vi "Differentiate 3D.vi"(0 "Timebase":dbl[](array[numeric]) format="%.2f", 3 "Sample Rate 4":dbl format="%.2f", 4 "Fixed Sample Rate":bool=TRUE, 5 "Data (in)":dbl[][](array[numeric]) format="%.2f") -> (2 "Data (differentiated)":dbl[][](graph))   [LabVIEW 2016]
uses:
  <vilib>/Analysis/2dsp.llb/Derivative x(t).vi
  <vilib>/Analysis/NI_AALPro.lvlib
panel:
  out "Data (differentiated) 2":dbl[][](graph)
  in  "Minimum TIme difference 1ms 4":dbl=0.001
  in  "Timebase 3":dbl[](array[numeric]) format="%.2f"
  in  "Minimum TIme difference 1ms 3":dbl=0.001
  in  "Sample Rate 3":dbl format="%.2f"
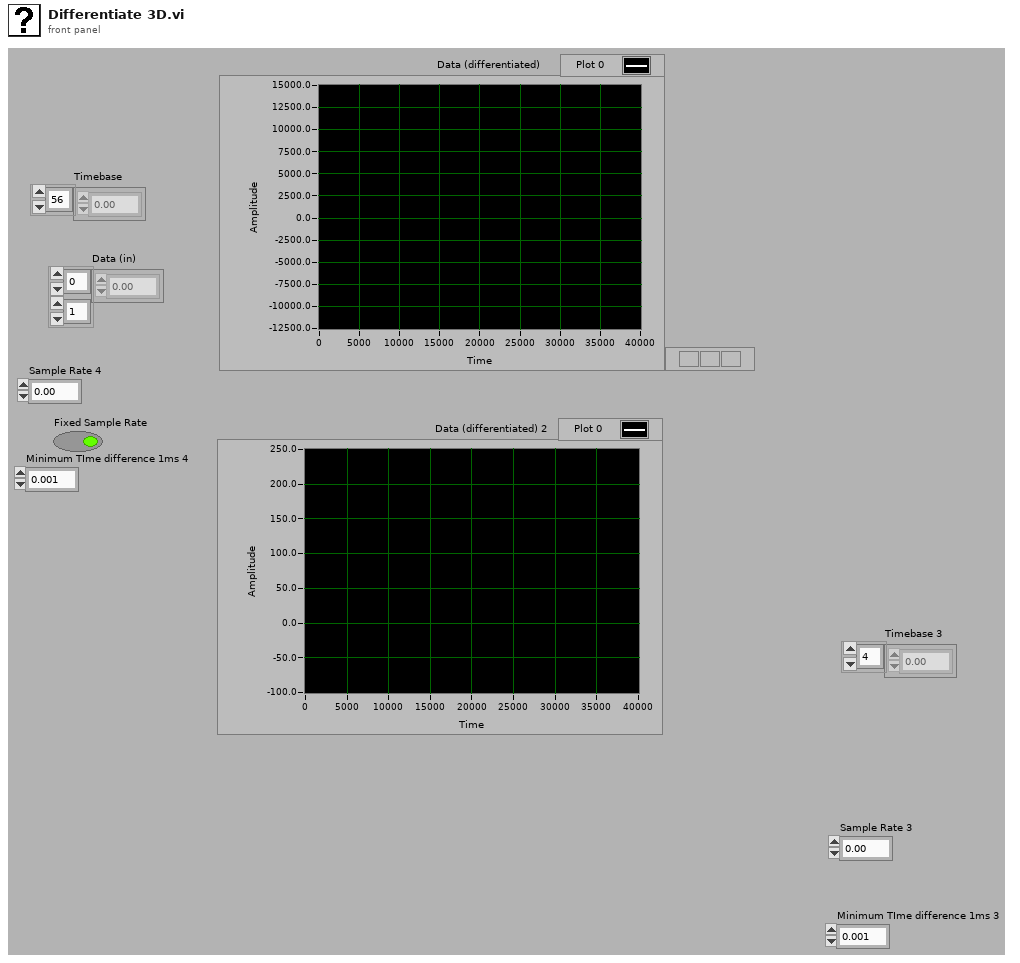
[diagram p1: front panel]
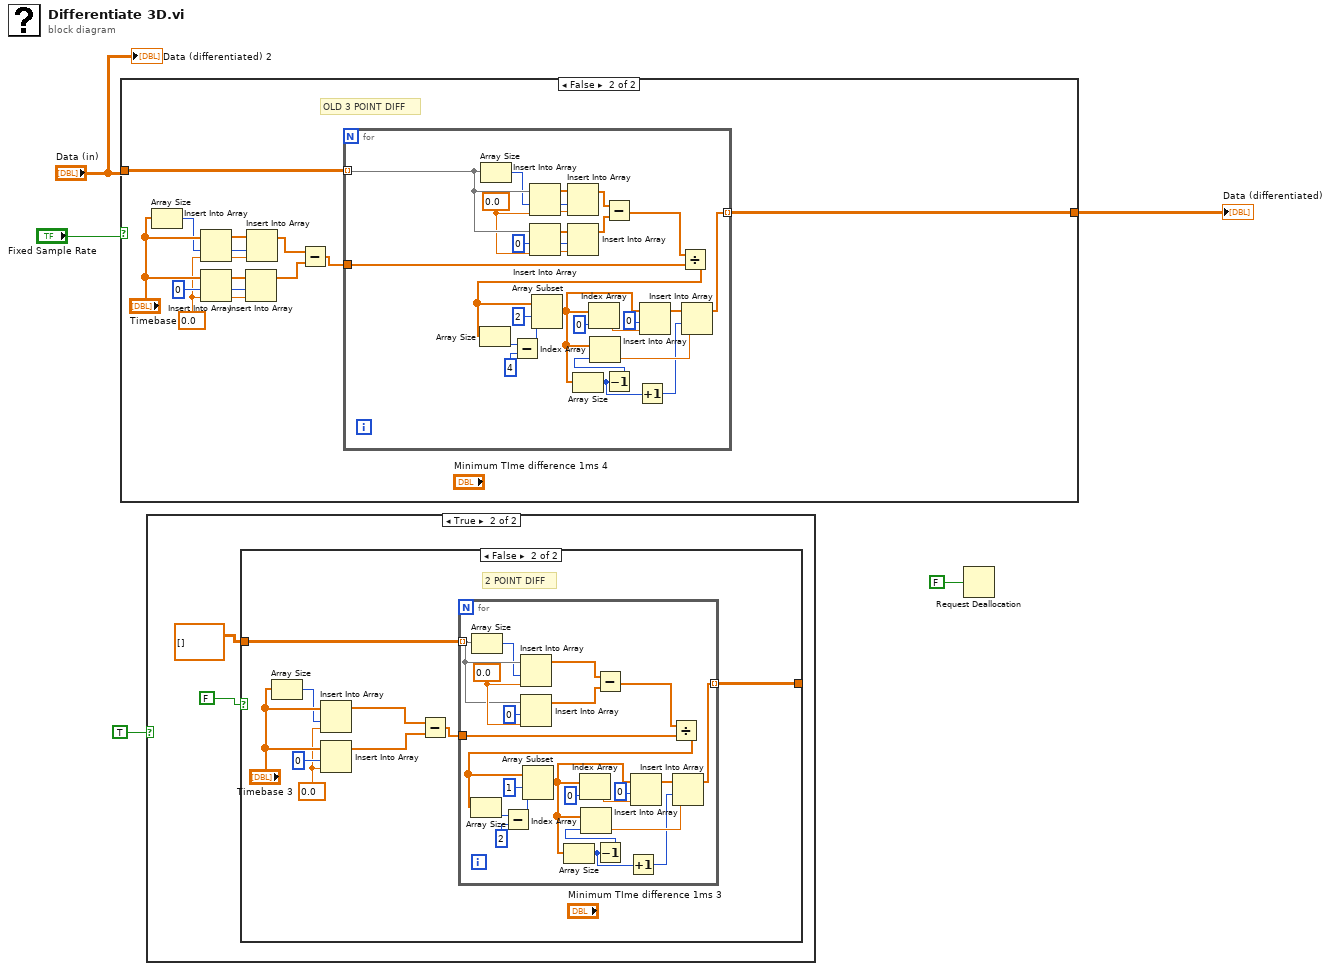
[diagram p0: block diagram]
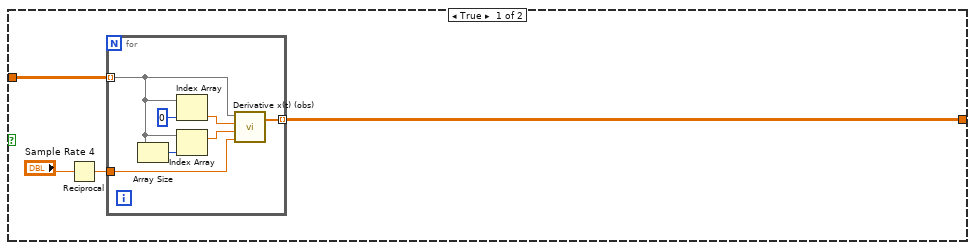
[diagram p2: hidden frame]
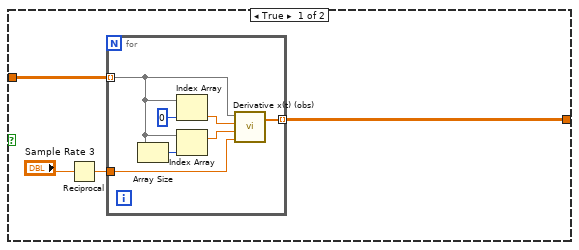
[diagram p4: hidden frame]
diagram:
  n1 = case shown="False" "Fixed Sample Rate" {
    tunnel: [w7 w19] -> w3
    tunnel: "Data (in)" -> [w6 w17]
    frame True {
      n2 = Reciprocal(x="Sample Rate 4") -> (1/x=w8:dbl)
      n3 = for {
        tunnel: w6 -> [w14] mode=indexing
        tunnel: w8 -> [w16]
        tunnel: [w10] -> w7 mode=indexing
        n4 = Array Size(array=w14) -> (size(s)=w13:i32)
        n5 = Index Array(array=w14, index=0 ("Index")) -> (element=w11:dbl)
        n6 = Index Array(array=w14, index=w13) -> (element=w12:dbl)
        n7 = call <vilib>:"Derivative x(t) (obs).vi"("dt"=w16, "final condition"=w12, "initial condition"=w11, "X"=w14) -> ("dX/dt"=w10:dbl[])  [unwired: 1 out]
      }
    }
    frame False {
      w21 = 0.0 ("new element/subarray")
      w24 = 0 ("index")
      # "OLD 3 POINT DIFF"
      n8 = Array Size(array="Timebase") -> (size(s)=w22:i32)
      n9 = Insert Into Array(array="Timebase", index=w22, new element=w21) -> (w23:dbl[])
      n10 = Insert Into Array(array="Timebase", index=w24, new element=w21) -> (w26:dbl[])
      n11 = Insert Into Array(array=w26, index=w24, new element=w21) -> (w25:dbl[])
      n12 = Insert Into Array(array=w23, index=w22, new element=w21) -> (w18:dbl[])
      n13 = Subtract(x=w18, y=w25) -> (x-y=w20:dbl[])
      n14 = for {
        tunnel: w17 -> [w50] mode=indexing
        tunnel: w20 -> [w52]
        tunnel: [w51] -> w19 mode=indexing
        w44 = 0.0 ("new element/subarray")
        w47 = 0 ("index")
        n15 = Array Size(array=w50) -> (size(s)=w29:i32)
        n16 = Insert Into Array(array=w50, index=w29, new element=w44) -> (w45:dbl[])
        n17 = Insert Into Array(array=w50, index=w47, new element=w44) -> (w49:dbl[])
        n18 = Insert Into Array(array=w45, index=w29, new element=w44) -> (w46:dbl[])
        n19 = Insert Into Array(array=w49, index=w47, new element=w44) -> (w48:dbl[])
        n20 = Subtract(x=w46, y=w48) -> (x-y=w28:dbl[])
        n21 = Divide(x=w28, y=w52) -> (x/y=w42:dbl[])
        n22 = Array Size(array=w42) -> (size(s)=w41:i32)
        n23 = Subtract(x=w41, y=4) -> (x-y=w39:i32)
        n24 = Array Subset(array=w42, index=2, length=w39) -> (w37:dbl[])
        n25 = Array Size(array=w37) -> (size(s)=w32:i32)
        n26 = Index Array(array=w37, index=0) -> (element=w35:dbl)
        n27 = Decrement(x=w32) -> (x-1=w33:i32)
        n28 = Index Array(array=w37, index=w33) -> (element=w34:dbl)
        n29 = Increment(x=w32) -> (x+1=w31:i32)
        n30 = Insert Into Array(array=w37, index=0, new element=w35) -> (w36:dbl[])
        n31 = Insert Into Array(array=w36, index=w31, new element=w34) -> (w51:dbl[])
      }
    }
  }
  "Data (differentiated)" <- w3
  n32 = case shown="True" TRUE {
    frame False {
    }
    frame True {
      n33 = case shown="False" FALSE {
        tunnel: [w56 w68] -> _
        tunnel: dbl[][] [] ("Data (in)") -> [w55 w74]
        frame True {
          n34 = Reciprocal(x="Sample Rate 3") -> (1/x=w57:dbl)
          n35 = for {
            tunnel: w55 -> [w63] mode=indexing
            tunnel: w57 -> [w65]
            tunnel: [w59] -> w56 mode=indexing
            n36 = Array Size(array=w63) -> (size(s)=w62:i32)
            n37 = Index Array(array=w63, index=0 ("Index")) -> (element=w60:dbl)
            n38 = Index Array(array=w63, index=w62) -> (element=w61:dbl)
            n39 = call <vilib>:"Derivative x(t) (obs).vi"("dt"=w65, "final condition"=w61, "initial condition"=w60, "X"=w63) -> ("dX/dt"=w59:dbl[])  [unwired: 1 out]
          }
        }
        frame False {
          w70 = 0.0 ("new element/subarray")
          # "2 POINT DIFF"
          n40 = Array Size(array="Timebase 3") -> (size(s)=w71:i32)
          n41 = Insert Into Array(array="Timebase 3", index=w71, new element=w70) -> (w67:dbl[])
          n42 = Insert Into Array(array="Timebase 3", index=0, new element=w70) -> (w66:dbl[])
          n43 = Subtract(x=w67, y=w66) -> (x-y=w69:dbl[])
          n44 = for {
            tunnel: w74 -> [w95] mode=indexing
            tunnel: w69 -> [w94]
            tunnel: [w77] -> w68 mode=indexing
            w96 = 0.0 ("new element/subarray")
            n45 = Array Size(array=w95) -> (size(s)=w79:i32)
            n46 = Insert Into Array(array=w95, index=w79, new element=w96) -> (w76:dbl[])
            n47 = Insert Into Array(array=w95, index=0, new element=w96) -> (w75:dbl[])
            n48 = Subtract(x=w76, y=w75) -> (x-y=w78:dbl[])
            n49 = Divide(x=w78, y=w94) -> (x/y=w92:dbl[])
            n50 = Array Size(array=w92) -> (size(s)=w91:i32)
            n51 = Subtract(x=w91, y=2) -> (x-y=w89:i32)
            n52 = Array Subset(array=w92, index=1, length=w89) -> (w87:dbl[])
            n53 = Array Size(array=w87) -> (size(s)=w82:i32)
            n54 = Index Array(array=w87, index=0) -> (element=w85:dbl)
            n55 = Decrement(x=w82) -> (x-1=w83:i32)
            n56 = Index Array(array=w87, index=w83) -> (element=w84:dbl)
            n57 = Increment(x=w82) -> (x+1=w81:i32)
            n58 = Insert Into Array(array=w87, index=0, new element=w85) -> (w86:dbl[])
            n59 = Insert Into Array(array=w86, index=w81, new element=w84) -> (w77:dbl[])
          }
        }
      }
    }
  }
  n60 = Request Deallocation(FALSE ("flag")) -> ()
  "Data (differentiated) 2" <- "Data (in)"
